vi "Init.vi"(8 "error in (no error)":errorcluster, 9 "Config File Path":path=path "", 10 "Name":string, 11 "Mock Log Handler In":refnum<class "Mock Log Handler.lvclass">) -> (0 "error out":errorcluster, 3 "Mock Log Handler Out":refnum<class "Mock Log Handler.lvclass">)   [LabVIEW 2020, in "Mock Log Handler.lvclass"]
doc: "Initialize the class and creates necessary references. Anything initialized here is released in the Clear.vi method."
uses:
  Framework/Base/Base.lvclass/Base.ctl
  <vilib>/Utility/file.llb/Application Directory.vi
  Mock Log Handler.lvclass
  Framework/Base/Base.lvclass
  Private/Log Entry.ctl
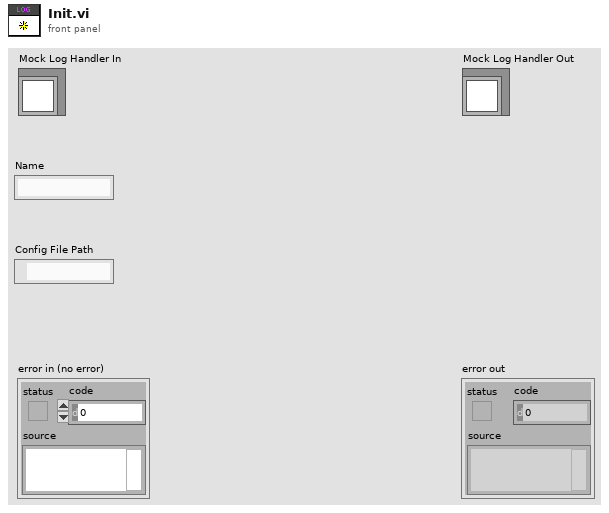
[diagram p1: front panel]
types:
  T1 = typedef "Mock Log Handler.lvclass/Log Entry.ctl" = cluster{"Level":string, "Source":string, "Message":string}
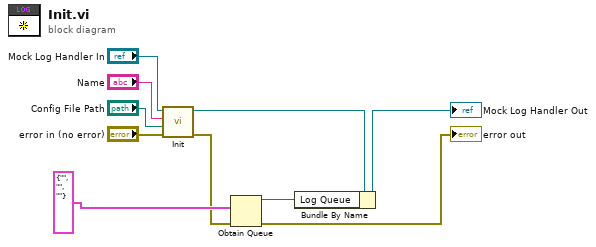
[diagram p0: block diagram]
diagram:
  n1 = call-parent "Init.vi"("error in (no error)"="error in (no error)", "Config File Path"="Config File Path", "Name"="Name", "Base In"="Mock Log Handler In") -> ("error out"=w2:errorcluster, "Base Out"=w10:refnum<class "Mock Log Handler.lvclass">)  [unwired: 6 in]
  n2 = Obtain Queue(element data type=T1 {"Level"="", "Source"="", "Message"=""}, error in (no error)=w2) -> (queue out=w3:refnum<queue>, error out=→"error out":errorcluster)  [unwired: 3 in, 1 out]
  n3 = Bundle By Name(cluster=w10, "Log Queue"=w3) -> (→"Mock Log Handler Out":refnum<class "Mock Log Handler.lvclass">)
